vi "AUTO_EVENTS_TRIGGER.vi"(8 "error in":errorcluster) -> (0 "error out":errorcluster, 2 "raw array":bool[](array[boolean]), 3 "Array":bool[](array[boolean]))   [LabVIEW 2017]
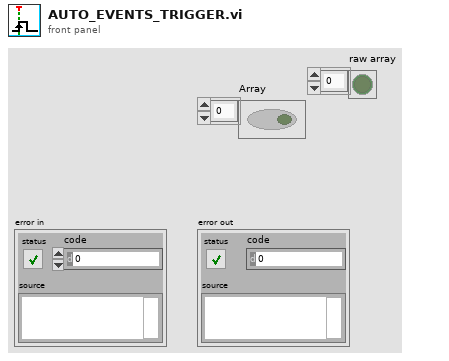
[diagram p1: front panel]
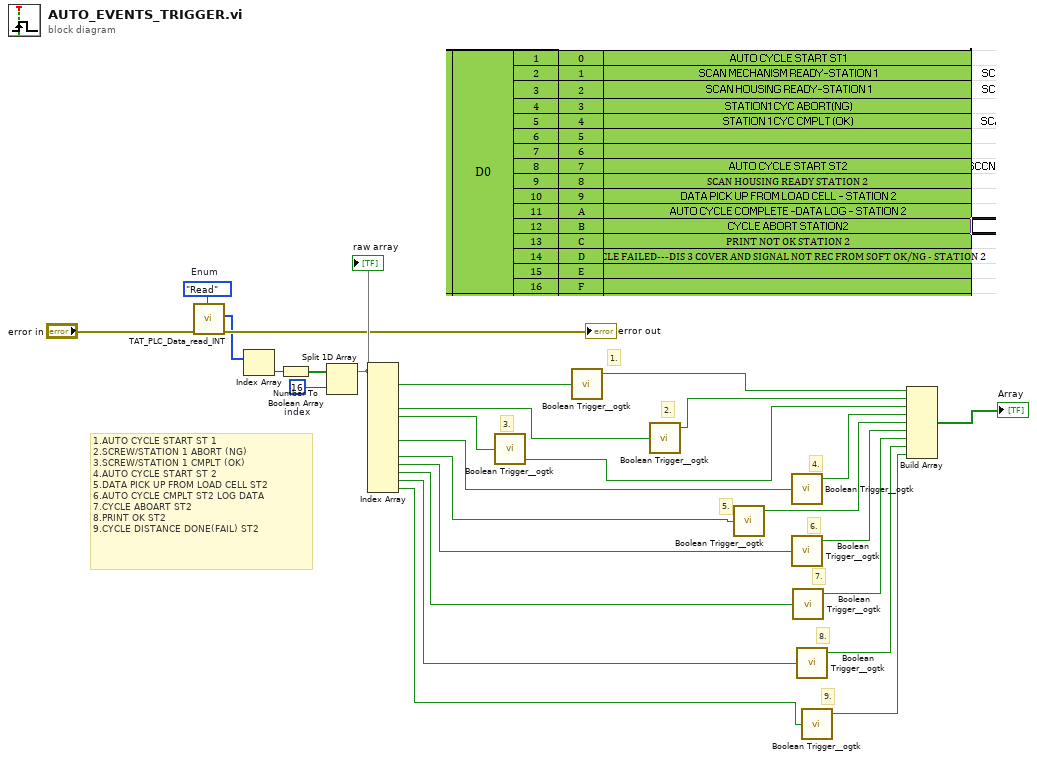
[diagram p0: block diagram]
diagram:
  w25 = 16  # index
  w20 = enum16{"Read", "Write"}."Read"  # Enum
  # "9."
  # "8."
  # "7."
  # "6."
  # "5."
  # "4."
  # "3."
  # "2."
  # "1."
  # "1.AUTO CYCLE START ST 1\n2.SCREW/STATION 1 ABORT (NG)\n3.SCREW/STATION 1 CMPLT (OK)\n4.AUTO CYCLE START ST 2\n5.DATA PICK UP FROM LOAD CELL ST2\n6.AUTO CYCLE CMPLT ST2 LOG DATA\n7.CYCLE ABOART ST2\n8.PRINT OK ST2\n9.CYCLE DISTANCE DONE(FAIL) ST2"
  n1 = call "TAT_PLC_Data_read_INT.vi"("Enum"=w20, "error in (no error)"="error in") -> ("error out"=→"error out":errorcluster, "Array 2"=w22:u16[])  [unwired: 8 in]
  n2 = Index Array(array=w22) -> (element=w23:u16)  [unwired: 1 in]
  n3 = Number To Boolean Array(number=w23) -> (Boolean array=w24:bool[])
  n4 = Split 1D Array(array=w24, index=w25) -> (first subarray=w27:bool[])  [unwired: 1 out]
  "raw array" <- w27
  n5 = Index Array(array=w27) -> (element #1=w19:bool, element #4=w17:bool, element #5=w9:bool, element #8=w8:bool, element #10=w7:bool, element #11=w6:bool, element #12=w5:bool, element #13=w2:bool, element #14=w1:bool)  [unwired: 14 in, 5 out]
  n6 = call <userlib>:"Boolean Trigger__ogtk.vi"("Boolean Input"=w9) -> ("Falling Edge"=w14:bool)  [unwired: 1 in, 1 out]
  n7 = call <userlib>:"Boolean Trigger__ogtk.vi"("Boolean Input"=w19) -> ("Rising Edge"=w11:bool)  [unwired: 1 in, 1 out]
  n8 = call <userlib>:"Boolean Trigger__ogtk.vi"("Boolean Input"=w17) -> ("Rising Edge"=w16:bool)  [unwired: 1 in, 1 out]
  n9 = call <userlib>:"Boolean Trigger__ogtk.vi"("Boolean Input"=w7) -> ("Rising Edge"=w13:bool)  [unwired: 1 in, 1 out]
  n10 = call <userlib>:"Boolean Trigger__ogtk.vi"("Boolean Input"=w8) -> ("Rising Edge"=w15:bool)  [unwired: 1 in, 1 out]
  n11 = call <userlib>:"Boolean Trigger__ogtk.vi"("Boolean Input"=w6) -> ("Rising Edge"=w12:bool)  [unwired: 1 in, 1 out]
  n12 = call <userlib>:"Boolean Trigger__ogtk.vi"("Boolean Input"=w5) -> ("Rising Edge"=w10:bool)  [unwired: 1 in, 1 out]
  n13 = call <userlib>:"Boolean Trigger__ogtk.vi"("Boolean Input"=w2) -> ("Rising Edge"=w4:bool)  [unwired: 1 in, 1 out]
  n14 = call <userlib>:"Boolean Trigger__ogtk.vi"("Boolean Input"=w1) -> ("Rising Edge"=w3:bool)  [unwired: 1 in, 1 out]
  n15 = Build Array(w11, w16, w14, w15, w13, w12, w10, w4, w3) -> (→"Array":bool[])
